vi "Add Private Key.vi"(8 "error in (no error)":errorcluster, 11 "Agent Fixture in":refnum<class "Agent Fixture.lvclass">) -> (0 "error out":errorcluster, 3 "Agent Fixture out":refnum<class "Agent Fixture.lvclass">)   [LabVIEW 2013, in "libssh2_integration_tests.lvlib" / "Agent Fixture.lvclass"]
uses:
  Agent Fixture.lvclass
  Agent Fixture.lvclass/Agent Fixture.ctl
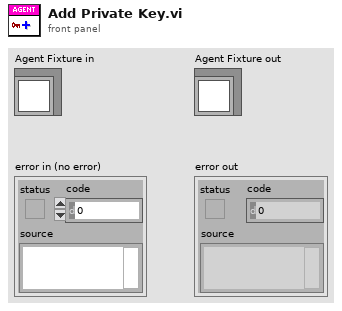
[diagram p1: front panel]
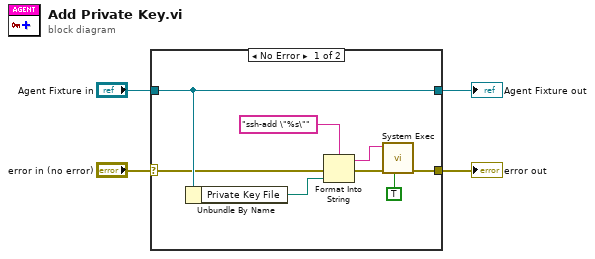
[diagram p0: block diagram]
diagram:
  n1 = case shown="No Error" "error in (no error)" {
    selector: "error in (no error)" -> [w7 w14]
    tunnel: [w11 w14] -> w3
    tunnel: [w10 w13] -> w1
    tunnel: "Agent Fixture in" -> [w10 w13]
    frame No Error {
      n2 = Unbundle By Name(w10) -> ("Private Key File"=w5:path)
      n3 = Format Into String(format string="ssh-add \"%s\"", error in=w7, w5) -> (resulting string=w8:string, error out=w6:errorcluster)  [unwired: 1 in]
      n4 = call <vilib>:"System Exec.vi"("run minimized? (F)"=TRUE, "error in (no error)"=w6, "command line"=w8) -> ("error out"=w11:errorcluster)  [unwired: 5 in, 3 out]
    }
    frame Error {
    }
  }
  "error out" <- w3
  "Agent Fixture out" <- w1
